vi "WSVCAP SHL FPGA LL I2C Write Data Lines.vi"(0 "Write Bit (U64)":u64, 11 "error in (no error)":errorcluster, 13 "Socket Mask":u64 format="%012x", 14 "UUT Set (0/1) (Legacy)":u8) -> (15 "error out":errorcluster)   [LabVIEW 2017]
uses:
  WSVCAP SHL FPGA LL I2C Debug Global.vi
  <vilib>/eio/EIONode/EIONode.xnode
  <vilib>/rvi/eio/common/nirviEmuTemplateMethod_errors.vi
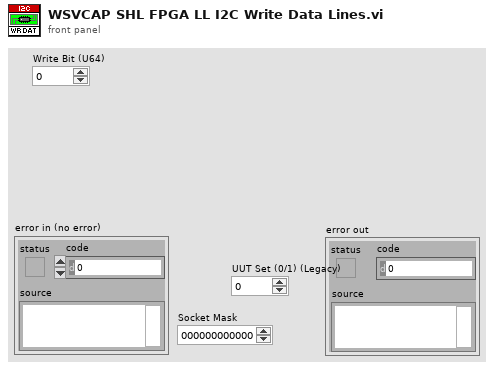
[diagram p1: front panel]
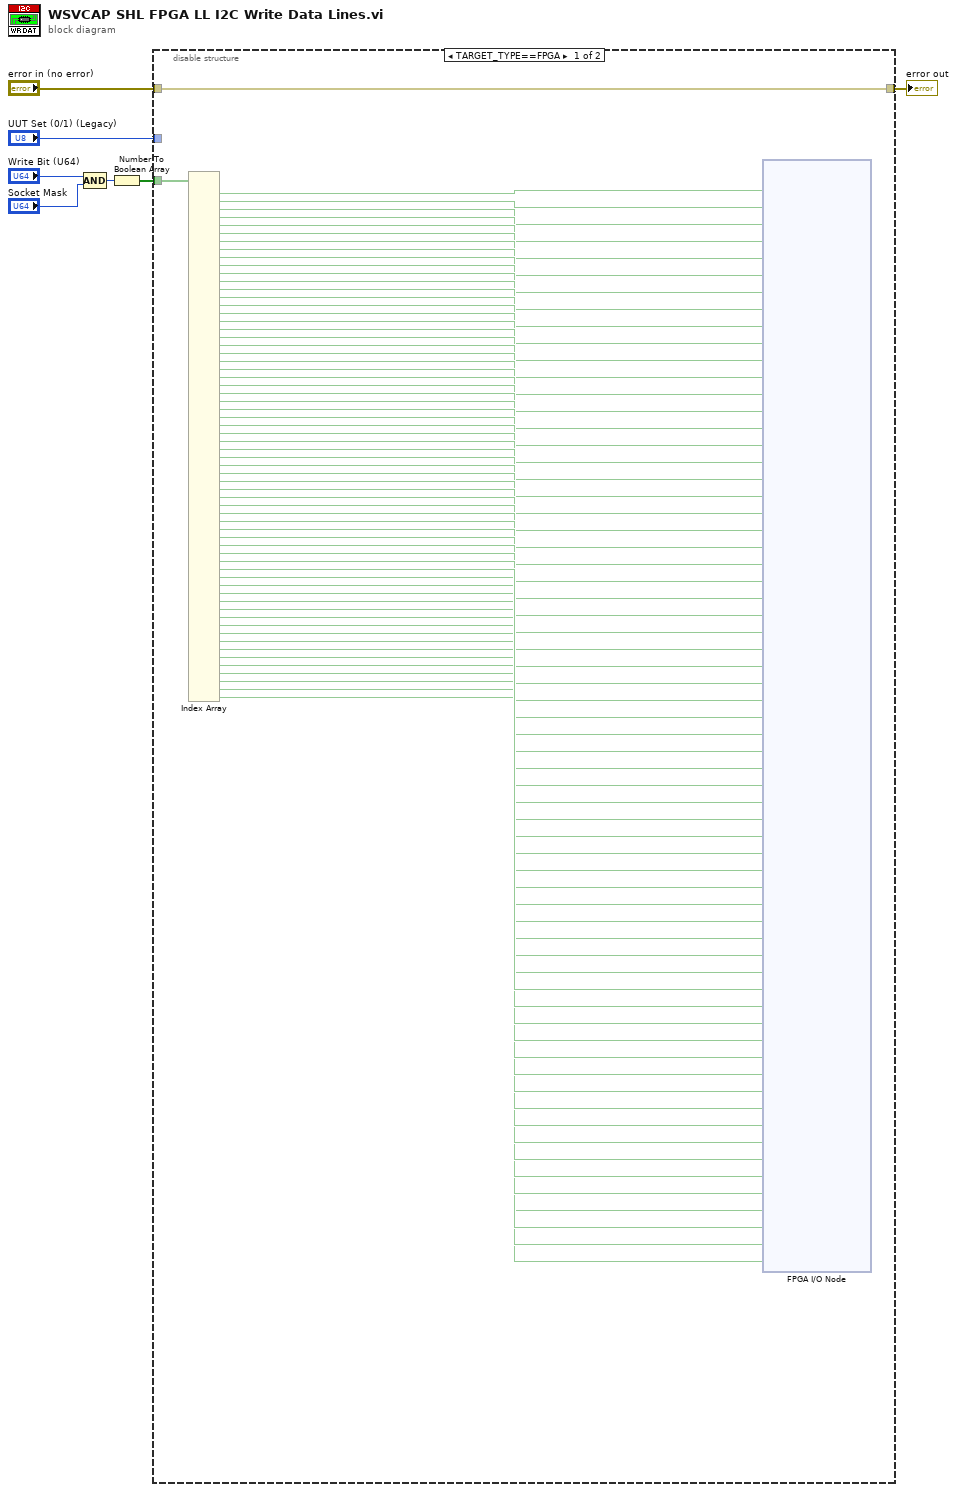
[diagram p0: block diagram]
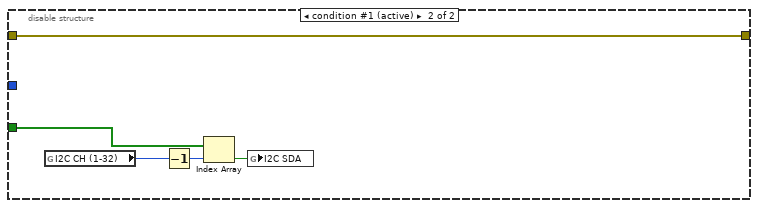
[diagram p2: hidden frame]
diagram:
  n1 = Compound Arithmetic op=AND("Write Bit (U64)", "Socket Mask") -> (w2:u64)
  n2 = Number To Boolean Array(number=w2) -> (Boolean array=w5:bool[])
  n3 = disable-structure shown="TARGET_TYPE==FPGA" {
    disable-tunnel: w5 -> [w24 w77]
    disable-tunnel: [w73 w78] -> w7
    disable-tunnel: "error in (no error)" -> [w73 w78]
    disable-tunnel: "UUT Set (0/1) (Legacy)" -> [_ _]
    frame condition #0 {
      n4 = Index Array(array=w24) -> (element #1=w25:bool, element #2=w26:bool, element #3=w27:bool, element #4=w28:bool, element #5=w29:bool, element #6=w30:bool, element #7=w31:bool, element #8=w32:bool, element #9=w33:bool, element #10=w34:bool, element #11=w35:bool, element #12=w36:bool, element #13=w37:bool, element #14=w38:bool, element #15=w39:bool, element #16=w40:bool, element #17=w41:bool, element #18=w42:bool, element #19=w43:bool, element #20=w44:bool, element #21=w45:bool, element #22=w46:bool, element #23=w47:bool, element #24=w48:bool, element #25=w49:bool, element #26=w50:bool, element #27=w51:bool, element #28=w52:bool, element #29=w53:bool, element #30=w54:bool, element #31=w55:bool, element #32=w56:bool, element #33=w57:bool, element #34=w58:bool, element #35=w59:bool, element #36=w60:bool, element #37=w61:bool, element #38=w62:bool, element #39=w63:bool, element #40=w64:bool, element #41=w65:bool, element #42=w66:bool, element #43=w67:bool, element #44=w68:bool, element #45=w69:bool, element #46=w70:bool, element #47=w71:bool, element #48=w72:bool, element #49=w23:bool, element #50=w22:bool, element #51=w21:bool, element #52=w20:bool, element #53=w19:bool, element #54=w18:bool, element #55=w17:bool, element #56=w16:bool, element #57=w15:bool, element #58=w14:bool, element #59=w13:bool, element #60=w12:bool, element #61=w10:bool, element #62=w11:bool, element #63=w9:bool, element #64=w8:bool)  [unwired: 64 in]
      n5 = xnode "FPGA I/O Node"("I2C_SDA_S1"=w25, "I2C_SDA_S2"=w26, "I2C_SDA_S3"=w27, "I2C_SDA_S4"=w28, "I2C_SDA_S5"=w29, "I2C_SDA_S6"=w30, "I2C_SDA_S7"=w31, "I2C_SDA_S8"=w32, "I2C_SDA_S9"=w33, "I2C_SDA_S10"=w34, "I2C_SDA_S11"=w35, "I2C_SDA_S12"=w36, "I2C_SDA_S13"=w37, "I2C_SDA_S14"=w38, "I2C_SDA_S15"=w39, "I2C_SDA_S16"=w40, "I2C_SDA_S17"=w41, "I2C_SDA_S18"=w42, "I2C_SDA_S19"=w43, "I2C_SDA_S20"=w44, "I2C_SDA_S21"=w45, "I2C_SDA_S22"=w46, "I2C_SDA_S23"=w47, "I2C_SDA_S24"=w48, "I2C_SDA_S25"=w49, "I2C_SDA_S26"=w50, "I2C_SDA_S27"=w51, "I2C_SDA_S28"=w52, "I2C_SDA_S29"=w53, "I2C_SDA_S30"=w54, "I2C_SDA_S31"=w55, "I2C_SDA_S32"=w56, "I2C_SDA_S33"=w57, "I2C_SDA_S34"=w58, "I2C_SDA_S35"=w59, "I2C_SDA_S36"=w60, "I2C_SDA_S37"=w61, "I2C_SDA_S38"=w62, "I2C_SDA_S39"=w63, "I2C_SDA_S40"=w64, "I2C_SDA_S41"=w65, "I2C_SDA_S42"=w66, "I2C_SDA_S43"=w67, "I2C_SDA_S44"=w68, "I2C_SDA_S45"=w69, "I2C_SDA_S46"=w70, "I2C_SDA_S47"=w71, "I2C_SDA_S48"=w72, "I2C_SDA_S49"=w23, "I2C_SDA_S50"=w22, "I2C_SDA_S51"=w21, "I2C_SDA_S52"=w20, "I2C_SDA_S53"=w19, "I2C_SDA_S54"=w18, "I2C_SDA_S55"=w17, "I2C_SDA_S56"=w16, "I2C_SDA_S57"=w15, "I2C_SDA_S58"=w14, "I2C_SDA_S59"=w13, "I2C_SDA_S60"=w12, "I2C_SDA_S61"=w10, "I2C_SDA_S62"=w11, "I2C_SDA_S63"=w9, "I2C_SDA_S64"=w8) -> ()  [unwired: 65 in, 65 out]
    }
    frame condition #1 (active) {
      n6 = global read "WSVCAP SHL FPGA LL I2C Debug Global.vi" "I2C CH (1-32)"() -> (w76:i32)
      n7 = Decrement(x=w76) -> (x-1=w74:i32)
      n8 = Index Array(array=w77, index=w74) -> (element=w75:bool)
      n9 = global write "WSVCAP SHL FPGA LL I2C Debug Global.vi" "I2C SDA"(w75) -> ()
    }
  }
  "error out" <- w7
